vi "check_access_done.vi"(8 "error in":errorcluster) -> (0 "error out":errorcluster, 3 "return":i32)   [LabVIEW 2016]
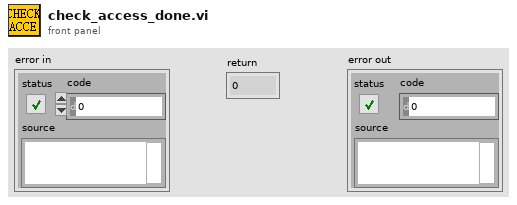
[diagram p1: front panel]
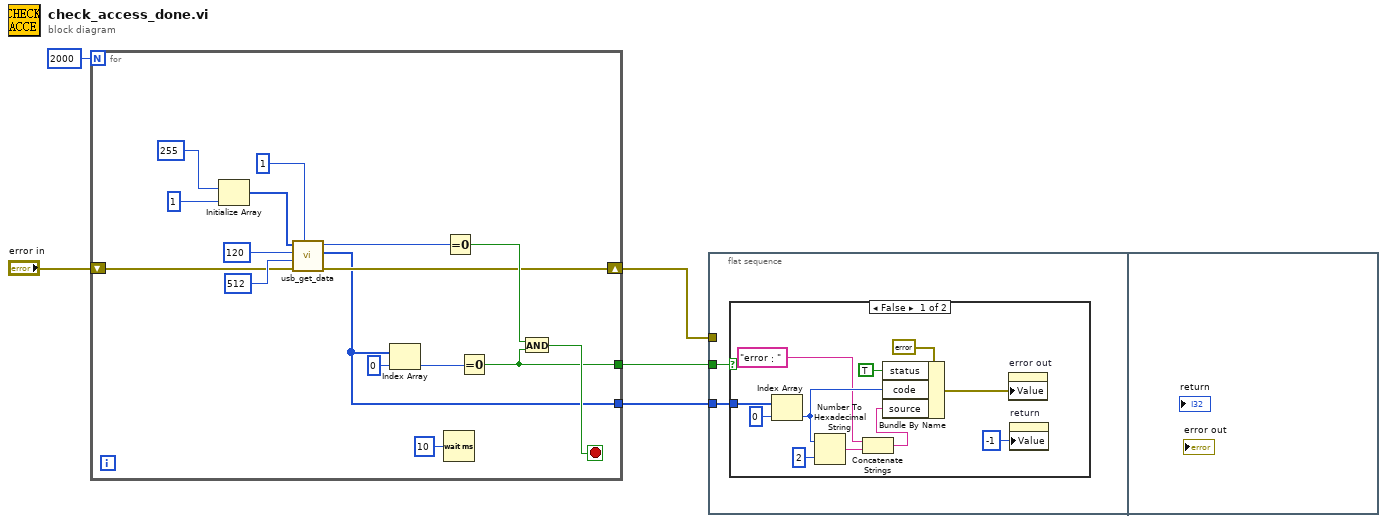
[diagram p0: block diagram]
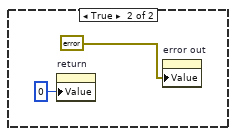
[diagram p2: hidden frame]
diagram:
  n1 = for {
    N: 2000 -> [_]
    tunnel: [w11] -> w3
    shift-right: [w8] -> w2
    shift-left: "error in" -> [w9]
    tunnel: [w6] -> w1
    stop <- w12 stop-if-true
    n2 = Initialize Array(u8 255 ("element"), 1 ("dimension size")) -> (w18:u8[])
    n3 = call "usb_get_data.vi"("byVdCmdHeaderLen"=u16 1, "error in"=w9, "I2C_VD_BUFFER_RW"=u16 512, "I2C_SLAVE_ID"=u8 120, "data"=w18) -> ("error out"=w8:errorcluster, "data out"=w6:u8[], "return"=w13:i32)  [unwired: 4 in]
    n4 = Index Array(array=w6, index=0) -> (element=w7:u8)
    n5 = Wait (ms)(milliseconds to wait=u32 10) -> ()  [unwired: 1 out]
    n6 = Equal To 0?(x=w13) -> (x = 0?=w10:bool)
    n7 = Equal To 0?(x=w7) -> (x = 0?=w11:bool)
    n8 = And(x=w10, y=w11) -> (x .and. y?=w12:bool)
  }
  n9 = flat-sequence {
    tunnel: w3 -> [w23]
    tunnel: w2 -> [_]
    tunnel: w1 -> [w22]
    frame #0 {
      n10 = case shown="False" w23 {
        tunnel: w22 -> [w32 _]
        frame False {
          n11 = Index Array(array=w32, index=0) -> (element=w28:u8)
          n12 = Number To Hexadecimal String(1:i16 2 ("width (-)"), 2:w28) -> (0:w27:string)
          n13 = Concatenate Strings("error：" ("string"), w27) -> (w25:string)
          n14 = Bundle By Name(cluster=errorcluster {"status"=TRUE, "code"=1111100000, "source"="ERR:i2c transfer status always busy!"} ("error out"), "status"=TRUE, "code"=w28, "source"=w25) -> (w24:errorcluster)
          n15 = property on="error out" class="Clust (strict)"("Value"=w24) -> ()  [unwired: 2 in, 2 out]
          n16 = property on="return" class="DigNum (strict)"("Value"=-1 ("return")) -> ()  [unwired: 2 in, 2 out]
        }
        frame True {
          n17 = property on="return" class="DigNum (strict)"("Value"=0 ("return")) -> ()  [unwired: 2 in, 2 out]
          n18 = property on="error out" class="Clust (strict)"("Value"=errorcluster {"status"=FALSE, "code"=0, "source"="successful"} ("error out")) -> ()  [unwired: 2 in, 2 out]
        }
      }
    }
    frame #1 {
    }
  }
